vi "Start_Idle_Elevator.vi"(8 "error in (no error)":errorcluster, 11 "Elevator in":T1) -> (0 "error out":errorcluster, 3 "Elevator out":T1)   [LabVIEW 2026]
uses:
  Controls/Motion_Status_Enum.ctl
  Controls/Door_Status_Enum.ctl
  Controls/Occupy_Status.ctl
  Controls/Floor_Status.ctl
  Controls/Car_Calls_Status.ctl
  Controls/Hall_Calls_Status.ctl
  Controls/Elevator_Status.ctl
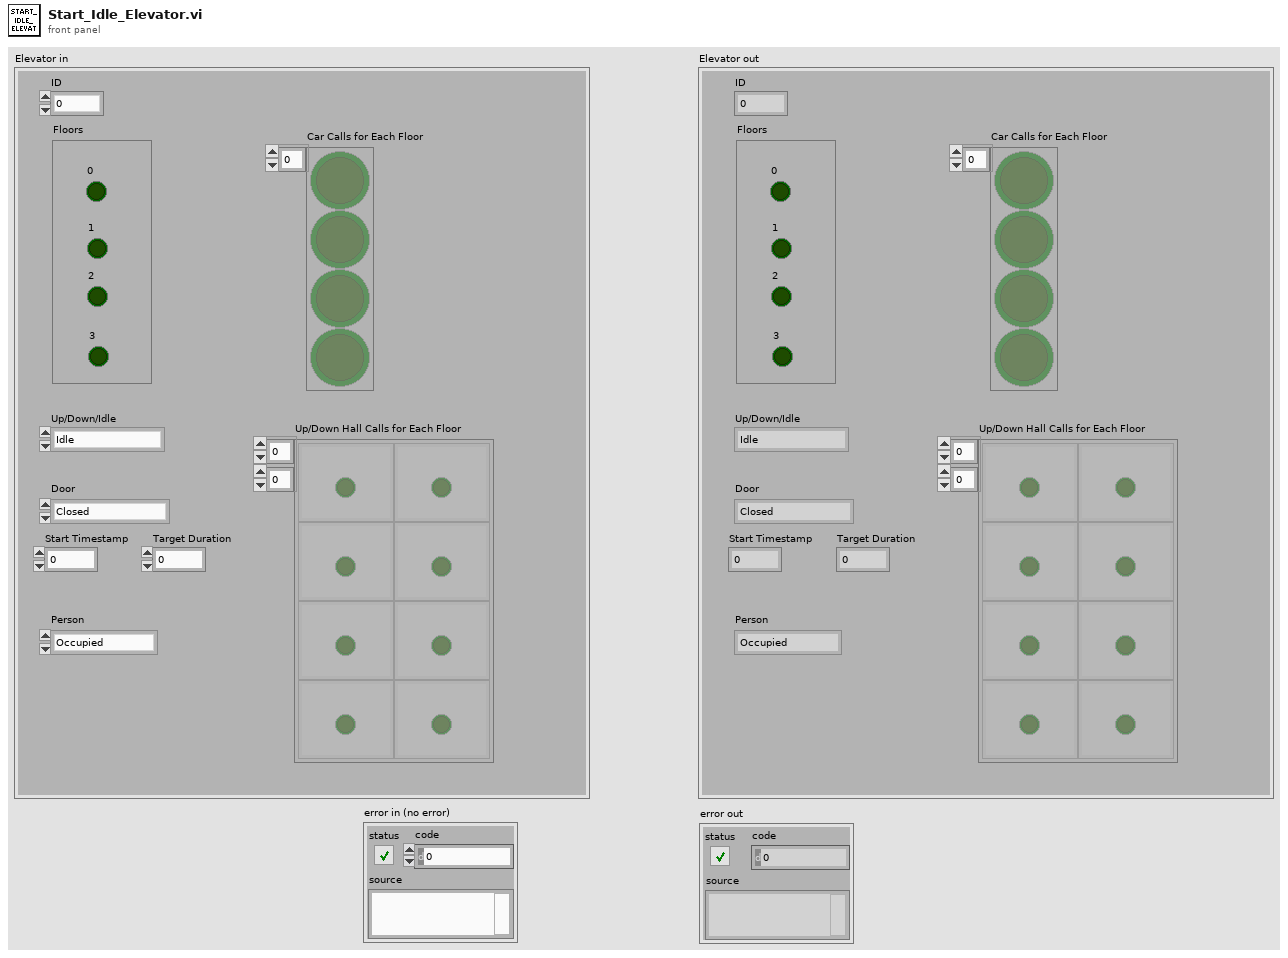
[diagram p1: front panel]
types:
  T1 = typedef "Elevator_Status.ctl" = cluster{"Door":T2, "Person":T3, "Floors":T4, "Up/Down/Idle":T5, "Car Calls for Each Floor":T6, "Up/Down Hall Calls for Each Floor":T7, "ID":i32, "Start Timestamp":u32, "Target Duration":dbl}
  T2 = typedef "Door_Status_Enum.ctl" = enum16{"Closed", "Open", "Opening", "Closing"}
  T3 = typedef "Occupy_Status.ctl" = enum16{"Occupied", "Empty"}
  T4 = typedef "Floor_Status.ctl" = cluster{"0":bool, "1":bool, "2":bool, "3":bool}
  T5 = typedef "Motion_Status_Enum.ctl" = enum16{"Idle", "Up", "Down"}
  T6 = typedef "Car_Calls_Status.ctl" = bool[]
  T7 = typedef "Hall_Calls_Status.ctl" = cluster{bool}[][]
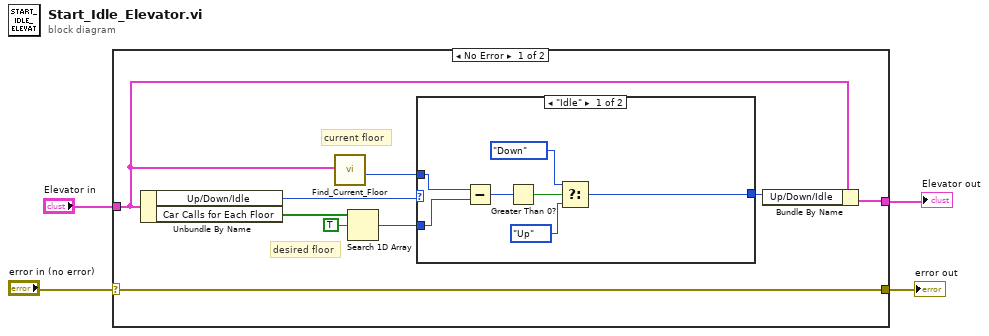
[diagram p0: block diagram]
diagram:
  n1 = case shown="No Error" "error in (no error)" {
    selector: "error in (no error)" -> [w5 w23]
    tunnel: [w8 w22] -> w4
    tunnel: "Elevator in" -> [w6 w22]
    tunnel: [w5 w23] -> w1
    frame No Error {
      # "desired floor"
      # "current floor"
      n2 = Unbundle By Name(w6) -> ("Up/Down/Idle"=w13:T5, "Car Calls for Each Floor"=w12:T6)
      n3 = call "Find_Current_Floor.vi"("Elevator Status in"=w6) -> ("Current Floor"=w7:i32)  [unwired: 7 in, 3 out]
      n4 = Search 1D Array(1D array=w12, element=TRUE) -> (index of element=w10:i32)  [unwired: 1 in]
      n5 = case shown="\"Idle\"" w13 {
        selector: w13 -> [_ w21]
        tunnel: w10 -> [w20 _]
        tunnel: [w15 w21] -> w9
        tunnel: w7 -> [w14 _]
        frame "Idle" {
          n6 = Subtract(x=w14, y=w20) -> (x-y=w19:i32)
          n7 = Greater Than 0?(x=w19) -> (x > 0?=w18:bool)
          n8 = Select(t=Motion_Status_Enum."Down" ("Up/Down/Idle"), s=w18, f=Motion_Status_Enum."Up" ("Up/Down/Idle")) -> (s? t:f=w15:T5)
        }
        frame Default {
        }
      }
      n9 = Bundle By Name(cluster=w6, "Up/Down/Idle"=w9) -> (w8:T1)
    }
    frame Error {
    }
  }
  "Elevator out" <- w4
  "error out" <- w1
